vi "InitKalman.vi"(0 "N_c":i32, 1 "Signal Avrage":dbl, 5 "N_r":i32, 7 "T":dbl, 9 "Alpha_c":dbl, 11 "Alpha_r":dbl, 12 "Signal":dbl[](array[numeric])) -> (3 "Init State":T3, 4 "Alpha_c out":dbl, 6 "Alpha_r out":dbl, 8 "P_n_1":T1, 10 "w_r_bar":dbl, 13 "Mesurement Noise Var":dbl, 14 "Init State Var":T2, 15 "w_ca_bar":dbl)   [LabVIEW 2012]
uses:
  <vilib>/Analysis/Matrix/Datatypes/RealMatrix.ctl
  <vilib>/Analysis/4window.llb/Hamming Window (DBL).vi
  <vilib>/Analysis/2dsp.llb/Real FFT.vi
  <vilib>/Analysis/NI_AALPro.lvlib
  <vilib>/Analysis/NI_AALBase.lvlib
  <vilib>/Analysis/Matrix/NI_Matrix.lvlib
panel:
  out "Harmanic Frequencies (a_r)":dbl[](array[numeric])
  out "Harmanic Frequencies":dbl[](array[numeric])
  out "a_r":dbl[](array[numeric])
  out "a_c":dbl[](array[numeric])
  out "output cluster":cluster{dbl[], dbl[]}(graph)
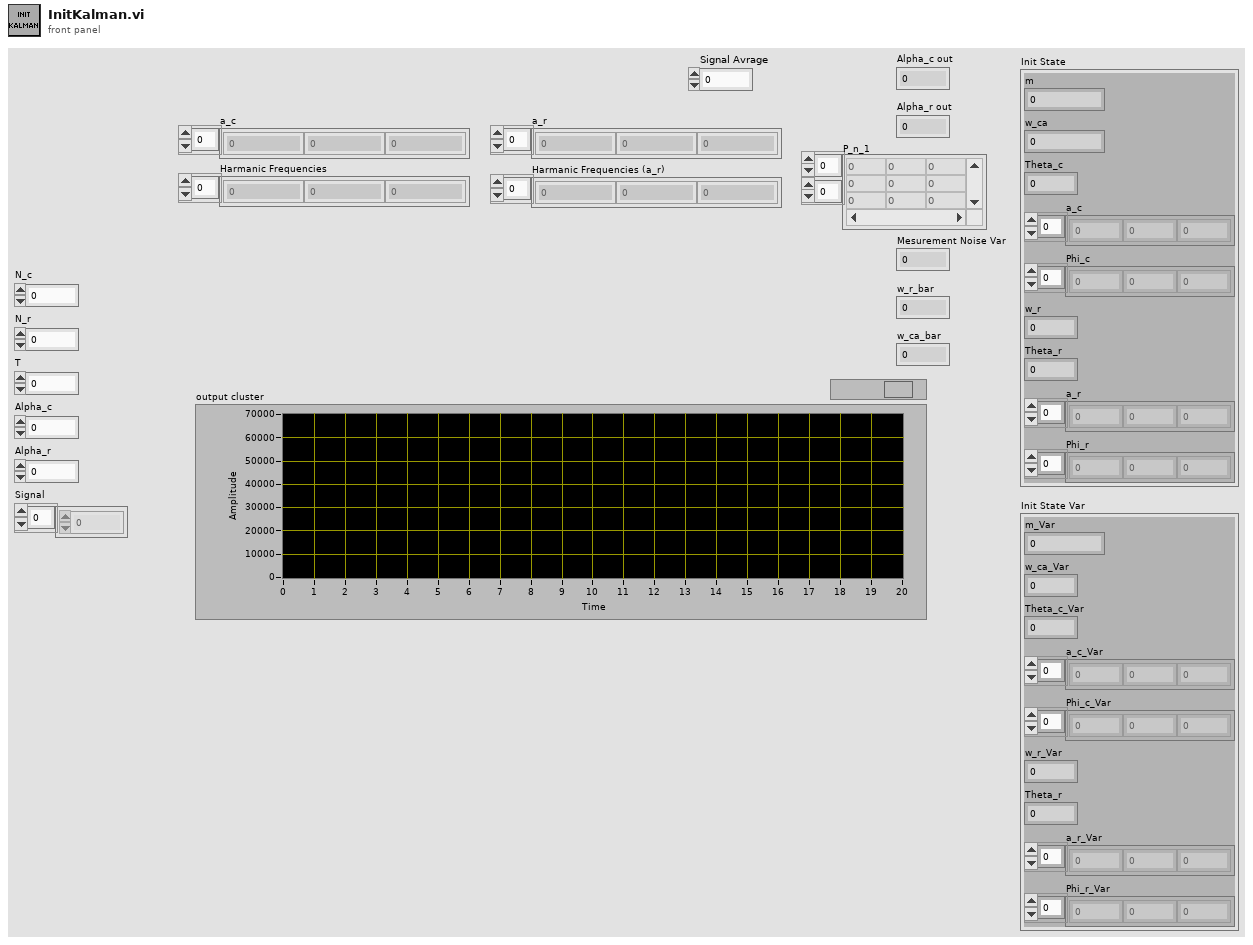
[diagram p1: front panel]
types:
  T1 = typedef "NI_Matrix.lvlib/RealMatrix.ctl" = dbl[][]
  T2 = cluster{"m_Var":dbl, "w_ca_Var":dbl, "Theta_c_Var":dbl, "a_c_Var":dbl[], "Phi_c_Var":dbl[], "w_r_Var":dbl, "Theta_r":dbl, "a_r_Var":dbl[], "Phi_r_Var":dbl[]}
  T3 = cluster{"m":dbl, "w_ca":dbl, "Theta_c":dbl, "a_c":dbl[], "Phi_c":dbl[], "w_r":dbl, "Theta_r":dbl, "a_r":dbl[], "Phi_r":dbl[]}
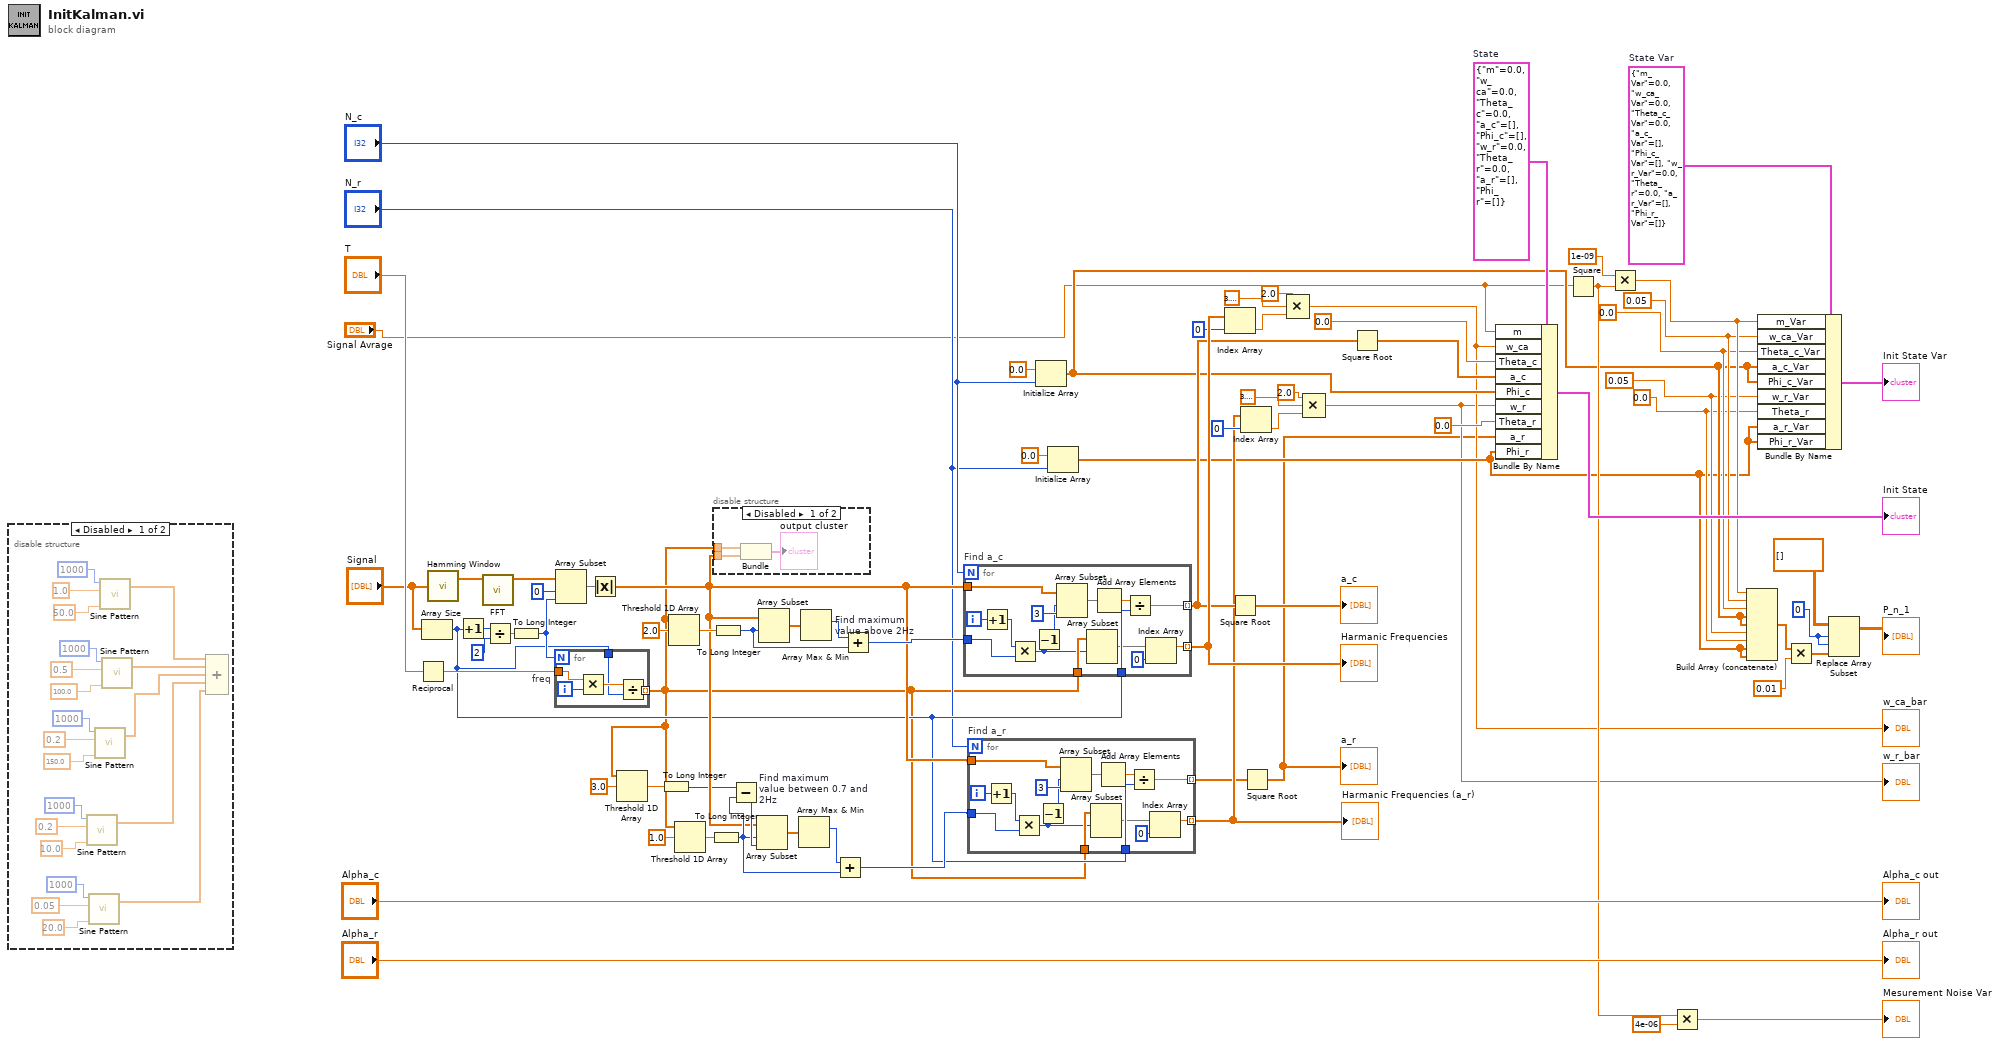
[diagram p0: block diagram]
diagram:
  w3 = 0
  w18 = 0.0 ("Theta_r")
  w19 = 0.05 ("w_r_Var")
  w21 = 0.0 ("Theta_c_Var")
  w22 = 0.05 ("w_ca_Var")
  w33 = T2 {"m_Var"=0.0, "w_ca_Var"=0.0, "Theta_c_Var"=0.0, "a_c_Var"=[], "Phi_c_Var"=[], "w_r_Var"=0.0, "Theta_r"=0.0, "a_r_Var"=[], "Phi_r_Var"=[]}  # State Var
  w52 = T3 {"m"=0.0, "w_ca"=0.0, "Theta_c"=0.0, "a_c"=[], "Phi_c"=[], "w_r"=0.0, "Theta_r"=0.0, "a_r"=[], "Phi_r"=[]}  # State
  n1 = disable-structure shown="Disabled" {
    frame Disabled {
      n2 = call <vilib>:"Sine Pattern.vi"("cycles"=10.0, "amplitude"=0.2, "samples"=1000) -> ("Sinusoidal Pattern"=w79:dbl[])  [unwired: 1 in, 1 out]
      n3 = call <vilib>:"Sine Pattern.vi"("cycles"=20.0, "amplitude"=0.05, "samples"=1000) -> ("Sinusoidal Pattern"=w78:dbl[])  [unwired: 1 in, 1 out]
      n4 = call <vilib>:"Sine Pattern.vi"("cycles"=150.0, "amplitude"=0.2, "samples"=1000) -> ("Sinusoidal Pattern"=w87:dbl[])  [unwired: 1 in, 1 out]
      n5 = call <vilib>:"Sine Pattern.vi"("cycles"=50.0, "amplitude"=1.0, "samples"=1000) -> ("Sinusoidal Pattern"=w86:dbl[])  [unwired: 1 in, 1 out]
      n6 = call <vilib>:"Sine Pattern.vi"("cycles"=100.0, "amplitude"=0.5, "samples"=1000) -> ("Sinusoidal Pattern"=w88:dbl[])  [unwired: 1 in, 1 out]
      n7 = Compound Arithmetic op=ADD(w86, w88, w87, w79, w78) -> ()  [unwired: 1 out]
    }
    frame Enabled {
    }
  }
  n8 = Reciprocal(x="T") -> (1/x=w70:dbl)
  n9 = Array Size(array="Signal") -> (size(s)=w53:i32)
  n10 = call-poly <vilib>:"Hamming Window.vi"("X"="Signal") -> ("Windowed X"=w77:dbl[])  [unwired: 1 out]
  n11 = Increment(x=w53) -> (x+1=w75:i32)
  n12 = call-poly <vilib>:"FFT.vi"("X"=w77) -> ("FFT {X}"=w76:cdb[])  [unwired: 9 in, 1 out]
  n13 = Divide(x=w75, y=2) -> (x/y=w73:dbl)
  n14 = To Long Integer(number=w73) -> (32bit integer=w68:i32)
  n15 = for "freq" {
    N: w68 -> [_]
    tunnel: w70 -> [w101]
    tunnel: [w98] -> w6 mode=indexing
    tunnel: w53 -> [w99]
    i -> [w102]
    n16 = Multiply(x=w101, y=w102) -> (x*y=w100:dbl)
    n17 = Divide(x=w100, y=w99) -> (x/y=w98:dbl)
  }
  n18 = Array Subset(array=w76, index=0, length=w68) -> (w71:cdb[])
  n19 = Absolute Value(x=w71) -> (abs(x)=w55:dbl[])
  n20 = Threshold 1D Array(2:3.0 ("threshold y"), 3:w6) -> (0:w8:dbl)  [unwired: 1 in]
  n21 = To Long Integer(number=w8) -> (32bit integer=w7:i32)
  n22 = Threshold 1D Array(2:2.0 ("threshold y"), 3:w6) -> (0:w66:dbl)  [unwired: 1 in]
  n23 = Threshold 1D Array(2:1.0 ("threshold y"), 3:w6) -> (0:w61:dbl)  [unwired: 1 in]
  n24 = To Long Integer(number=w61) -> (32bit integer=w56:i32)
  n25 = To Long Integer(number=w66) -> (32bit integer=w59:i32)
  n26 = disable-structure shown="Disabled" {
    disable-tunnel: w55 -> [w104 _]
    disable-tunnel: w6 -> [w103 _]
    frame Disabled {
      n27 = Bundle(w103, w104) -> (→"output cluster":cluster{dbl[], dbl[]})  [unwired: 1 in]
    }
    frame Enabled {
    }
  }
  n28 = Subtract(x=w7, y=w56) -> (x-y=w58:i32)
  n29 = Array Subset(array=w55, index=w56, length=w58) -> (w62:dbl[])
  n30 = Array Subset(array=w55, index=w59) -> (w65:dbl[])  [unwired: 1 in]
  n31 = Array Max & Min "Find maximum\nvalue between 0.7 and 2Hz"(array=w62) -> (max index (indices)=w57:i32)  [unwired: 3 out]
  n32 = Array Max & Min "Find maximum\nvalue above 2Hz"(array=w65) -> (max index (indices)=w64:i32)  [unwired: 3 out]
  n33 = Add(x=w57, y=w56) -> (x+y=w54:i32)
  n34 = Add(x=w64, y=w59) -> (x+y=w63:i32)
  n35 = for "Find a_c" {
    N: "N_c" -> [_]
    tunnel: w63 -> [w108]
    tunnel: w55 -> [w119]
    tunnel: w53 -> [w116]
    tunnel: [w114] -> w45 mode=indexing
    tunnel: w6 -> [w113]
    tunnel: [w111] -> w51 mode=indexing
    i -> [w115]
    n36 = Increment(x=w115) -> (x+1=w109:i32)
    n37 = Multiply(x=w109, y=w108) -> (x*y=w107:i32)
    n38 = Decrement(x=w107) -> (x-1=w106:i32)
    n39 = Array Subset(array=w119, index=w106, length=3) -> (w118:dbl[])
    n40 = Array Subset(array=w113, index=w107) -> (w112:dbl[])  [unwired: 1 in]
    n41 = Add Array Elements(numeric array=w118) -> (sum=w117:dbl)
    n42 = Divide(x=w117, y=w116) -> (x/y=w114:dbl)
    n43 = Index Array(array=w112, index=0) -> (element=w111:dbl)
  }
  "Harmanic Frequencies" <- w51
  n44 = for "Find a_r" {
    N: "N_r" -> [_]
    tunnel: w54 -> [w123]
    tunnel: w55 -> [w134]
    tunnel: w53 -> [w131]
    tunnel: [w129] -> w36 mode=indexing
    tunnel: w6 -> [w128]
    tunnel: [w126] -> w38 mode=indexing
    i -> [w130]
    n45 = Increment(x=w130) -> (x+1=w124:i32)
    n46 = Multiply(x=w124, y=w123) -> (x*y=w122:i32)
    n47 = Decrement(x=w122) -> (x-1=w121:i32)
    n48 = Array Subset(array=w134, index=w121, length=3) -> (w133:dbl[])
    n49 = Array Subset(array=w128, index=w122) -> (w127:dbl[])  [unwired: 1 in]
    n50 = Add Array Elements(numeric array=w133) -> (sum=w132:dbl)
    n51 = Divide(x=w132, y=w131) -> (x/y=w129:dbl)
    n52 = Index Array(array=w127, index=0) -> (element=w126:dbl)
  }
  "Harmanic Frequencies (a_r)" <- w38
  n53 = Initialize Array(0.0 ("element"), "N_c") -> (w20:dbl[])
  n54 = Initialize Array(0.0 ("element"), "N_r") -> (w17:dbl[])
  n55 = Index Array(array=w51, index=0) -> (element=w49:dbl)
  n56 = Square Root(x=w45) -> (sqrt(x)=→"a_c":dbl[])
  n57 = Index Array(array=w38, index=0) -> (element=w40:dbl)
  n58 = Square Root(x=w36) -> (sqrt(x)=w11:dbl[])
  "a_r" <- w11
  n59 = Compound Arithmetic op=MULTIPLY(2.0 ("value"), 3.141592653589793 ("value"), w49) -> (w14:dbl)
  "w_ca_bar" <- w14
  n60 = Compound Arithmetic op=MULTIPLY(2.0 ("value"), 3.141592653589793 ("value"), w40) -> (w13:dbl)
  "w_r_bar" <- w13
  n61 = Square Root(x=w45) -> (sqrt(x)=w44:dbl[])
  n62 = Bundle By Name(cluster=w52, "m"="Signal Avrage", "w_ca"=w14, "Theta_c"=0.0, "a_c"=w44, "Phi_c"=w20, "w_r"=w13, "Theta_r"=0.0, "a_r"=w11, "Phi_r"=w17) -> (→"Init State":T3)
  n63 = Square(x="Signal Avrage") -> (x^2=w26:dbl)
  n64 = Multiply(x=1e-09 ("y"), y=w26) -> (x*y=w23:dbl)
  n65 = Multiply(x=w26, y=4e-06) -> (x*y=→"Mesurement Noise Var":dbl)
  n66 = Build Array (concatenate)(w23, w22, w21, w20, w20, w19, w18, w17, w17) -> (w16:dbl[])
  n67 = Bundle By Name(cluster=w33, "m_Var"=w23, "w_ca_Var"=w22, "Theta_c_Var"=w21, "a_c_Var"=w20, "Phi_c_Var"=w20, "w_r_Var"=w19, "Theta_r"=w18, "a_r_Var"=w17, "Phi_r_Var"=w17) -> (→"Init State Var":T2)
  n68 = Multiply(x=w16, y=0.01) -> (x*y=w4:dbl[])
  n69 = Replace Array Subset(array=T1 [] ("matrix"), new element=w4, index (row)=w3, index (col)=w3) -> (→"P_n_1":T1)
  "Alpha_c out" <- "Alpha_c"
  "Alpha_r out" <- "Alpha_r"
